vi "Teleop.vi"   [LabVIEW 2016]
doc: "This VI is called for each TeleOp packet received from the DS where the robot is not disabled. It is often used to read from the joysticks and update I/O or to update setpoints for timed control loops. It should complete and return within 20 milliseconds or it may miss DS packets."
uses:
  <vilib>/Rock Robotics/WPI/Utilities/WPI_GetSetVariantRefNum.vi
  External/2ndContollerStatus.vi
  External/External.lvlib
types:
  T1 = enum16{"A", "B", "X", "Y", "LB", "RB", "Back", "Start"}
  T2 = typedef "WPI_JoystickDevRef.ctl" = cluster{"Device":T3}
  T3 = typedef "WPI_JoystickDeviceEnum.ctl" = enum16{"USB 0", "USB 1", "USB 2", "USB 3", "USB 4", "USB 5"}
  T4 = typedef "WPI_RobotDriveDevRef.ctl" = cluster{"DevStatus":errorcluster, "Motors[]":T5[], "Square Inputs":bool, "Max Output":dbl}
  T5 = typedef "WPI_MotorControlDeviceRef.ctl" = cluster{"DeviceStatus":errorcluster, "Type":T6, "PWM":cluster{"PWM Channel":T7, "DeadBand":T8}, "CAN":cluster{"Device Number":u8, "SetOutput VI Ref":variant, "GetOutput VI Ref":variant, "Enable VI Ref":variant, "Disable VI Ref":variant, "Data":variant}, "Invert":bool}
  T6 = typedef "WPI_MotorControlType.ctl" = enum16{"PWM", "CAN"}
  T7 = typedef "FPGA_DIOPWMChannel.ctl" = enum8{"PWM 0", "PWM 1", "PWM 2", "PWM 3", "PWM 4", "PWM 5", "PWM 6", "PWM 7", "PWM 8", "PWM 9", "PWM MXP 0", "PWM MXP 1", "PWM MXP 2", "PWM MXP 3", "PWM MXP 4", "PWM MXP 5", "PWM MXP 6", "PWM MXP 7", "PWM MXP 8", "PWM MXP 9", "Invalid"}
  T8 = typedef "WPI_PWMDeadband.ctl" = cluster{"Name":string, "maxPositivePwm":i32, "minPositivePwm":i32, "centerPwm":i32, "maxNegativePwm":i32, "minNegativePwm":i32, "angularRange":u16}
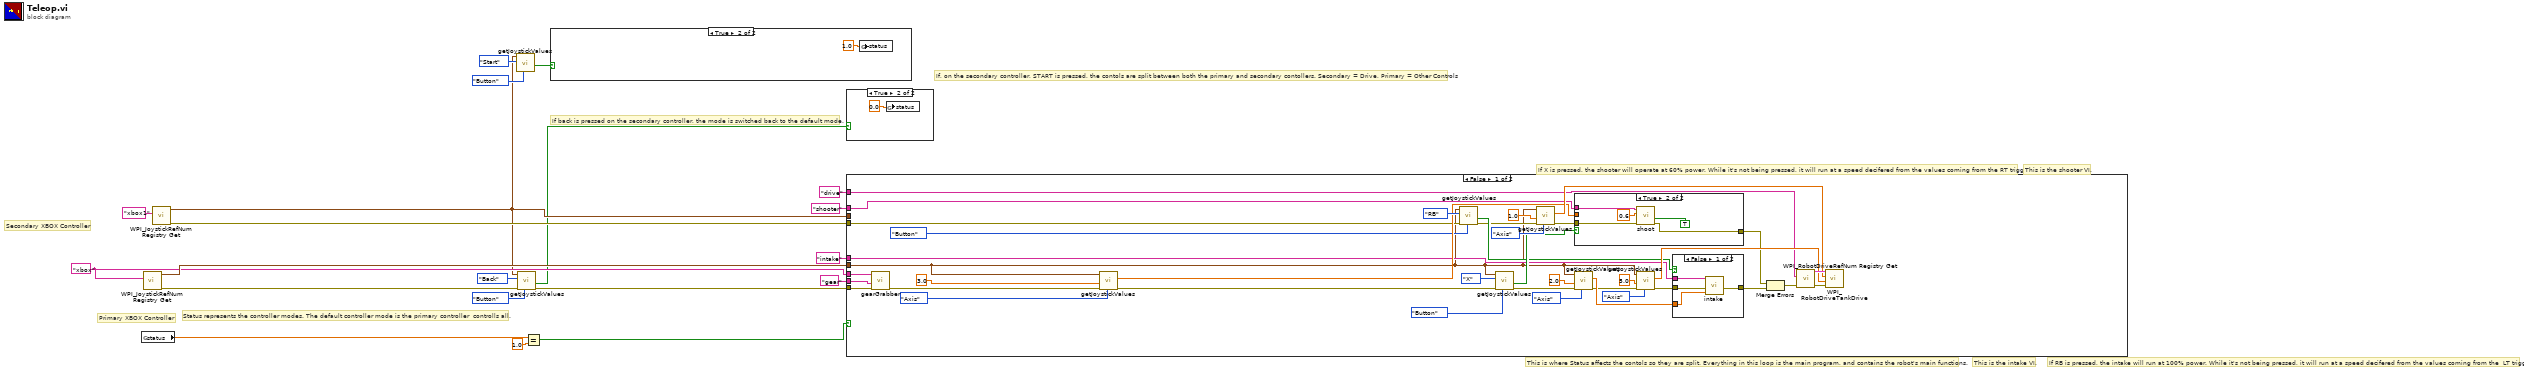
[diagram p0: block diagram]
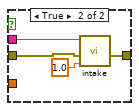
[diagram p4: hidden frame]
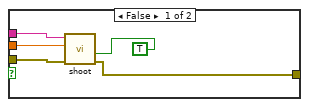
[diagram p5: hidden frame]
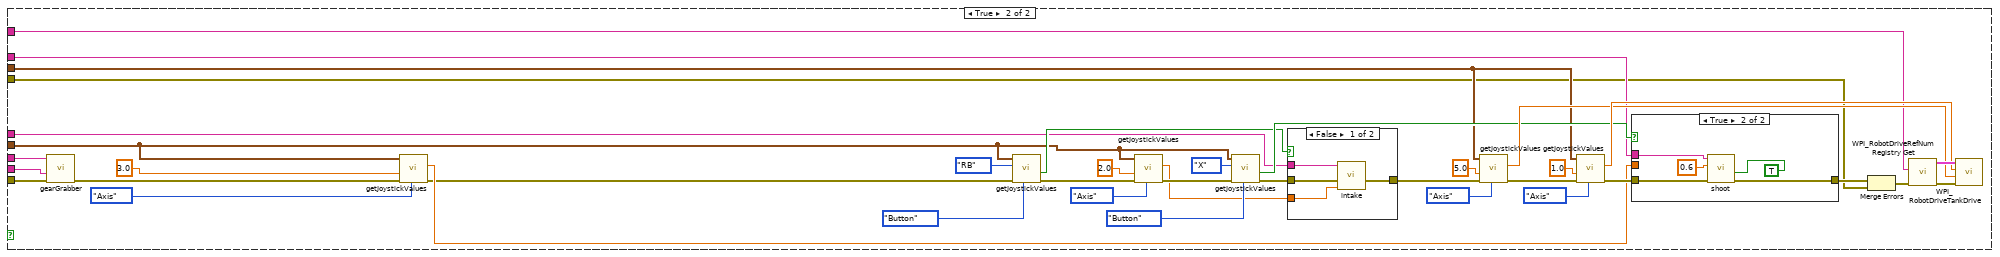
[diagram p6: hidden frame]
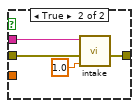
[diagram p7: hidden frame]
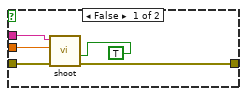
[diagram p8: hidden frame]
diagram:
  w15 = "xbox" ("xbox")
  # "This is the shooter VI."
  # "This is the intake VI."
  # "This is where Status affects the contols so they are split. Everything in this loop is the main program, and contains the robot's main functions."
  # "If RB is pressed, the intake will run at 100% power. While it's not being pressed, it will run at a speed decifered from the values coming from the  LT trigger."
  # "If X is pressed, the shooter will operate at 60% power. While it's not being pressed, it will run at a speed decifered from the values coming from the RT trigger."
  # "Secondary XBOX Controller"
  # "Primary XBOX Controller"
  # "If back is pressed on the secondary controller, the mode is switched back to the default mode."
  # "If, on the secondary controller, START is pressed, the contols are split between both the primary and secondary contollers. Secondary = Drive, Primary = Other Controls"
  # "Status represents the controller modes. The default controller mode is the primary controller  controlls all."
  n1 = global read "2ndContollerStatus.vi" "status"() -> (w3:dbl)
  n2 = call <vilib>:"WPI_JoystickRefNum Registry Get.vi"("refnum name"=w15) -> ("error out"=w5:errorcluster, "JoystickDevRef"=w20:T2)  [unwired: 9 in]
  n3 = call <vilib>:"WPI_JoystickRefNum Registry Get.vi"("refnum name"="xbox1" ("xbox1")) -> ("error out"=w18:errorcluster, "JoystickDevRef"=w7:T2)  [unwired: 9 in]
  n4 = call "getJoystickValues.vi"("Mode"=enum16{"Axis", "Button"}."Button", "buttonType"=T1."Start", "JoystickDevRef"=w7) -> ("Button Pressed"=w16:bool)  [unwired: 5 in, 3 out]
  n5 = call "getJoystickValues.vi"("Mode"=enum16{"Axis", "Button"}."Button", "error in (no error)"=w5, "buttonType"=T1."Back", "JoystickDevRef"=w7) -> ("error out"=w4:errorcluster, "Button Pressed"=w6:bool)  [unwired: 4 in, 2 out]
  n6 = Equal?(x=w3, y=1.0) -> (x = y?=w1:bool)
  n7 = case shown="True" w16 {
    frame False {
    }
    frame True {
      n8 = global write "2ndContollerStatus.vi" "status"(1.0 ("status")) -> ()
    }
  }
  n9 = case shown="True" w6 {
    frame False {
    }
    frame True {
      n10 = global write "2ndContollerStatus.vi" "status"(0.0 ("status")) -> ()
    }
  }
  n11 = case shown="False" w1 {
    tunnel: w20 -> [w25 w79]
    tunnel: w7 -> [_ w98]
    tunnel: w18 -> [w29 w85]
    tunnel: w15 -> [w40 w96]
    tunnel: "gear" ("gear") -> [w39 w95]
    tunnel: "intake" ("intake") -> [w37 w94]
    tunnel: "shooter" ("shooter") -> [w38 w93]
    tunnel: "drive" ("drive") -> [w36 w92]
    tunnel: w4 -> [w35 w91]
    frame False {
      n12 = call "gearGrabber.vi"("error in (no error)"=w35, "gear"=w39, "xbox"=w40) -> ("error out"=w34:errorcluster)  [unwired: 8 in]
      n13 = call "getJoystickValues.vi"("Mode"=enum16{"Axis", "Button"}."Axis", "error in (no error)"=w34, "Axis"=3.0, "JoystickDevRef"=w25) -> ("error out"=w33:errorcluster, "Value"=w43:dbl)  [unwired: 4 in, 2 out]
      n14 = call "getJoystickValues.vi"("Mode"=enum16{"Axis", "Button"}."Button", "error in (no error)"=w29, "buttonType"=enum16{"A", "B", "X", "Y", "LB", "RB"}."RB", "JoystickDevRef"=w25) -> ("error out"=w32:errorcluster, "Button Pressed"=w46:bool)  [unwired: 4 in, 2 out]
      n15 = call "getJoystickValues.vi"("Mode"=enum16{"Axis", "Button"}."Button", "error in (no error)"=w33, "buttonType"=enum16{"A", "B", "X", "Y", "LB", "RB"}."X", "JoystickDevRef"=w25) -> ("error out"=w24:errorcluster, "Button Pressed"=w53:bool)  [unwired: 4 in, 2 out]
      n16 = call "getJoystickValues.vi"("Mode"=enum16{"Axis", "Button"}."Axis", "error in (no error)"=w32, "Axis"=1.0, "JoystickDevRef"=w25) -> ("error out"=w51:errorcluster, "Value"=w56:dbl)  [unwired: 4 in, 2 out]
      n17 = case shown="True" w53 {
        tunnel: w51 -> [w73 w78]
        tunnel: [w72 w77] -> w50
        tunnel: w43 -> [w70 _]
        tunnel: w38 -> [w69 w74]
        frame False {
          n18 = call "shoot.vi"("Shooting Activated"=TRUE, "error in (no error)"=w73, "Motor Power"=w70, "refnum name"=w69) -> ("error out"=w72:errorcluster)  [unwired: 7 in]
        }
        frame True {
          n19 = call "shoot.vi"("Shooting Activated"=TRUE, "error in (no error)"=w78, "Motor Power"=0.6, "refnum name"=w74) -> ("error out"=w77:errorcluster)  [unwired: 7 in]
        }
      }
      n20 = call "getJoystickValues.vi"("Mode"=enum16{"Axis", "Button"}."Axis", "error in (no error)"=w24, "Axis"=2.0, "JoystickDevRef"=w25) -> ("error out"=w23:errorcluster, "Value"=w27:dbl)  [unwired: 4 in, 2 out]
      n21 = call "getJoystickValues.vi"("Mode"=enum16{"Axis", "Button"}."Axis", "error in (no error)"=w23, "Axis"=5.0, "JoystickDevRef"=w25) -> ("error out"=w30:errorcluster, "Value"=w55:dbl)  [unwired: 4 in, 2 out]
      n22 = case shown="False" w46 {
        tunnel: w30 -> [w64 w68]
        tunnel: [w63 w67] -> w31
        tunnel: w37 -> [w62 w65]
        tunnel: w27 -> [w61 _]
        frame False {
          n23 = call "intake.vi"("intakeSpeed"=w61, "error in (no error)"=w64, "intake"=w62) -> ("error out"=w63:errorcluster)  [unwired: 8 in]
        }
        frame True {
          n24 = call "intake.vi"("intakeSpeed"=1.0 ("intake speed"), "error in (no error)"=w68, "intake"=w65) -> ("error out"=w67:errorcluster)  [unwired: 8 in]
        }
      }
      n25 = Merge Errors(w50, w31) -> (w41:errorcluster)
      n26 = call <vilib>:"WPI_RobotDriveRefNum Registry Get.vi"("error in (no error)"=w41, "refnum name"=w36) -> ("error out"=w59:errorcluster, "RobotDriveDevRef"=w60:T4)  [unwired: 8 in]
      n27 = call <vilib>:"WPI_RobotDriveTankDrive.vi"("error in (no error)"=w59, "Right axis value"=w55, "Left axis value"=w56, "RobotDriveDevRef"=w60) -> ()  [unwired: 5 in, 3 out]
    }
    frame True {
      n28 = call "gearGrabber.vi"("error in (no error)"=w91, "gear"=w95, "xbox"=w96) -> ("error out"=w90:errorcluster)  [unwired: 8 in]
      n29 = call "getJoystickValues.vi"("Mode"=enum16{"Axis", "Button"}."Axis", "error in (no error)"=w90, "Axis"=3.0, "JoystickDevRef"=w79) -> ("error out"=w86:errorcluster, "Value"=w100:dbl)  [unwired: 4 in, 2 out]
      n30 = call "getJoystickValues.vi"("Mode"=enum16{"Axis", "Button"}."Button", "error in (no error)"=w86, "buttonType"=enum16{"A", "B", "X", "Y", "LB", "RB"}."RB", "JoystickDevRef"=w79) -> ("error out"=w84:errorcluster, "Button Pressed"=w103:bool)  [unwired: 4 in, 2 out]
      n31 = call "getJoystickValues.vi"("Mode"=enum16{"Axis", "Button"}."Axis", "error in (no error)"=w84, "Axis"=2.0, "JoystickDevRef"=w79) -> ("error out"=w83:errorcluster, "Value"=w82:dbl)  [unwired: 4 in, 2 out]
      n32 = call "getJoystickValues.vi"("Mode"=enum16{"Axis", "Button"}."Button", "error in (no error)"=w83, "buttonType"=enum16{"A", "B", "X", "Y", "LB", "RB"}."X", "JoystickDevRef"=w79) -> ("error out"=w89:errorcluster, "Button Pressed"=w110:bool)  [unwired: 4 in, 2 out]
      n33 = case shown="False" w103 {
        tunnel: w89 -> [w121 w125]
        tunnel: [w120 w124] -> w88
        tunnel: w94 -> [w119 w122]
        tunnel: w82 -> [w118 _]
        frame False {
          n34 = call "intake.vi"("intakeSpeed"=w118, "error in (no error)"=w121, "intake"=w119) -> ("error out"=w120:errorcluster)  [unwired: 8 in]
        }
        frame True {
          n35 = call "intake.vi"("intakeSpeed"=1.0 ("intake speed"), "error in (no error)"=w125, "intake"=w122) -> ("error out"=w124:errorcluster)  [unwired: 8 in]
        }
      }
      n36 = call "getJoystickValues.vi"("Mode"=enum16{"Axis", "Button"}."Axis", "error in (no error)"=w88, "Axis"=5.0, "JoystickDevRef"=w98) -> ("error out"=w87:errorcluster, "Value"=w112:dbl)  [unwired: 4 in, 2 out]
      n37 = call "getJoystickValues.vi"("Mode"=enum16{"Axis", "Button"}."Axis", "error in (no error)"=w87, "Axis"=1.0, "JoystickDevRef"=w98) -> ("error out"=w108:errorcluster, "Value"=w113:dbl)  [unwired: 4 in, 2 out]
      n38 = case shown="True" w110 {
        tunnel: w108 -> [w130 w135]
        tunnel: [w129 w134] -> w107
        tunnel: w100 -> [w127 _]
        tunnel: w93 -> [w126 w131]
        frame False {
          n39 = call "shoot.vi"("Shooting Activated"=TRUE, "error in (no error)"=w130, "Motor Power"=w127, "refnum name"=w126) -> ("error out"=w129:errorcluster)  [unwired: 7 in]
        }
        frame True {
          n40 = call "shoot.vi"("Shooting Activated"=TRUE, "error in (no error)"=w135, "Motor Power"=0.6, "refnum name"=w131) -> ("error out"=w134:errorcluster)  [unwired: 7 in]
        }
      }
      n41 = Merge Errors(w107, w85) -> (w97:errorcluster)
      n42 = call <vilib>:"WPI_RobotDriveRefNum Registry Get.vi"("error in (no error)"=w97, "refnum name"=w92) -> ("error out"=w116:errorcluster, "RobotDriveDevRef"=w117:T4)  [unwired: 8 in]
      n43 = call <vilib>:"WPI_RobotDriveTankDrive.vi"("error in (no error)"=w116, "Right axis value"=w112, "Left axis value"=w113, "RobotDriveDevRef"=w117) -> ()  [unwired: 5 in, 3 out]
    }
  }
